vi "VB.vi"() -> ()   [LabVIEW 2010]
panel:
  in  "stop":bool
  # "Алгоритм управления"
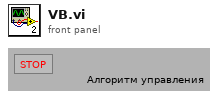
[diagram p1: front panel]
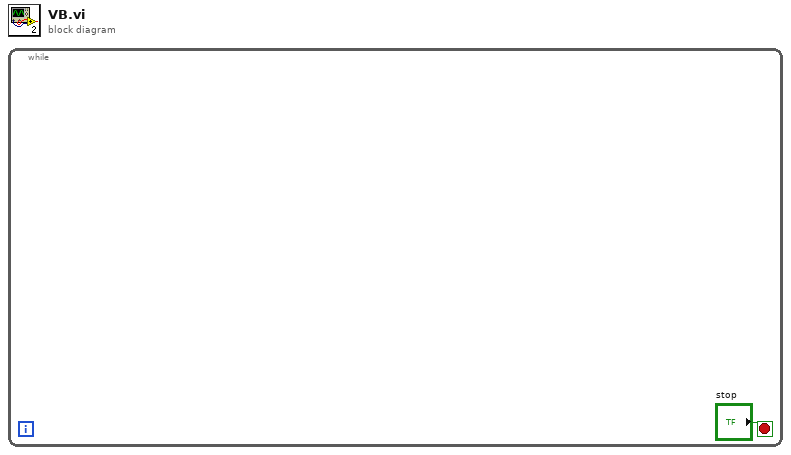
[diagram p0: block diagram]
diagram:
  n1 = while {
    stop <- "stop" stop-if-true
  }
